vi "Dequeue.vi"(6 "timeout in ms (-1)":i32=-1, 8 "error in (no error)":errorcluster, 11 "Message Queue":T2) -> (0 "error out":errorcluster, 1 "Message Data":variant, 2 "State":T3=enum."Initialize", 3 "Message Queue dub":T2, 4 "# elements in queue":i32, 5 "Caller Info":T1)   [LabVIEW 2019, in "Test.lvlib"]
doc: "This VI pulls messages off the Message Queue."
uses:
  Test.lvlib
  State Name.ctl
  Support/Shared/TypeDefs/Message Queue Ref.ctl
  85968e22-cec5-4834-9408-c5f0918d029d.vi
  0e969a01-278a-410f-94a4-bde872eff04a.vi
  <vilib>/Utility/error.llb/Clear Errors.vi
  <vilib>/Utility/error.llb/Error Cluster From Error Code.vi
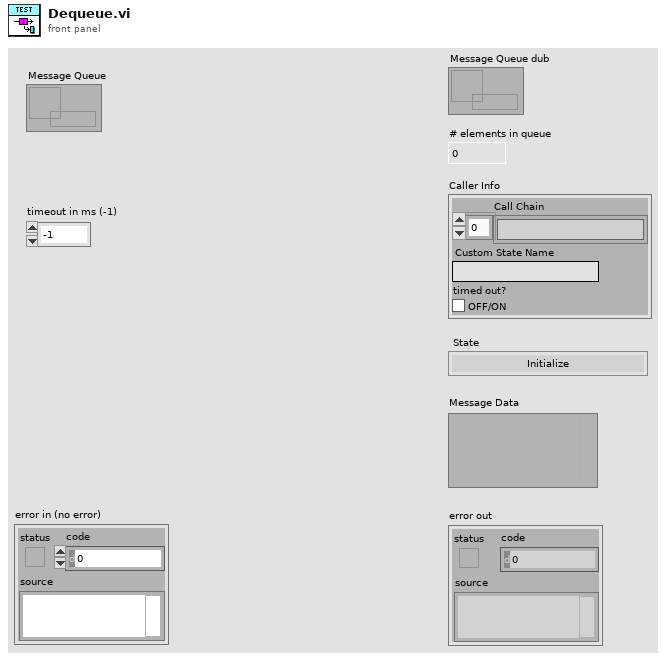
[diagram p1: front panel]
types:
  T1 = cluster{"Call Chain":string[], "Custom State Name":string, "timed out?":bool}
  T2 = typedef "Message Queue Ref.ctl" = refnum<queue>
  T3 = typedef "Test.lvlib/State Name.ctl" = enum16{"Default", "Initialize", "Re-Initialize", "Initialize Data", "Initialize Panel", "[Event Structure] Update Data", "Error", "Exit"}
  T4 = enum16{"Default", "Show FP", "Hide FP", "New Data", "Get Data"}
  T5 = cluster{"Module":string, "State Name":string, "State Dequeue Time":string, "Interval":string, "Call Chain":string, "# elements in queue":i32}
  T6 = cluster{"Call Chain":string[], "Desired State Name":string, "timed out?":bool}
  T7 = cluster{"Custom State Name":string, "Defined State Name":variant, "Call Chain":string[], "Message Data":variant}
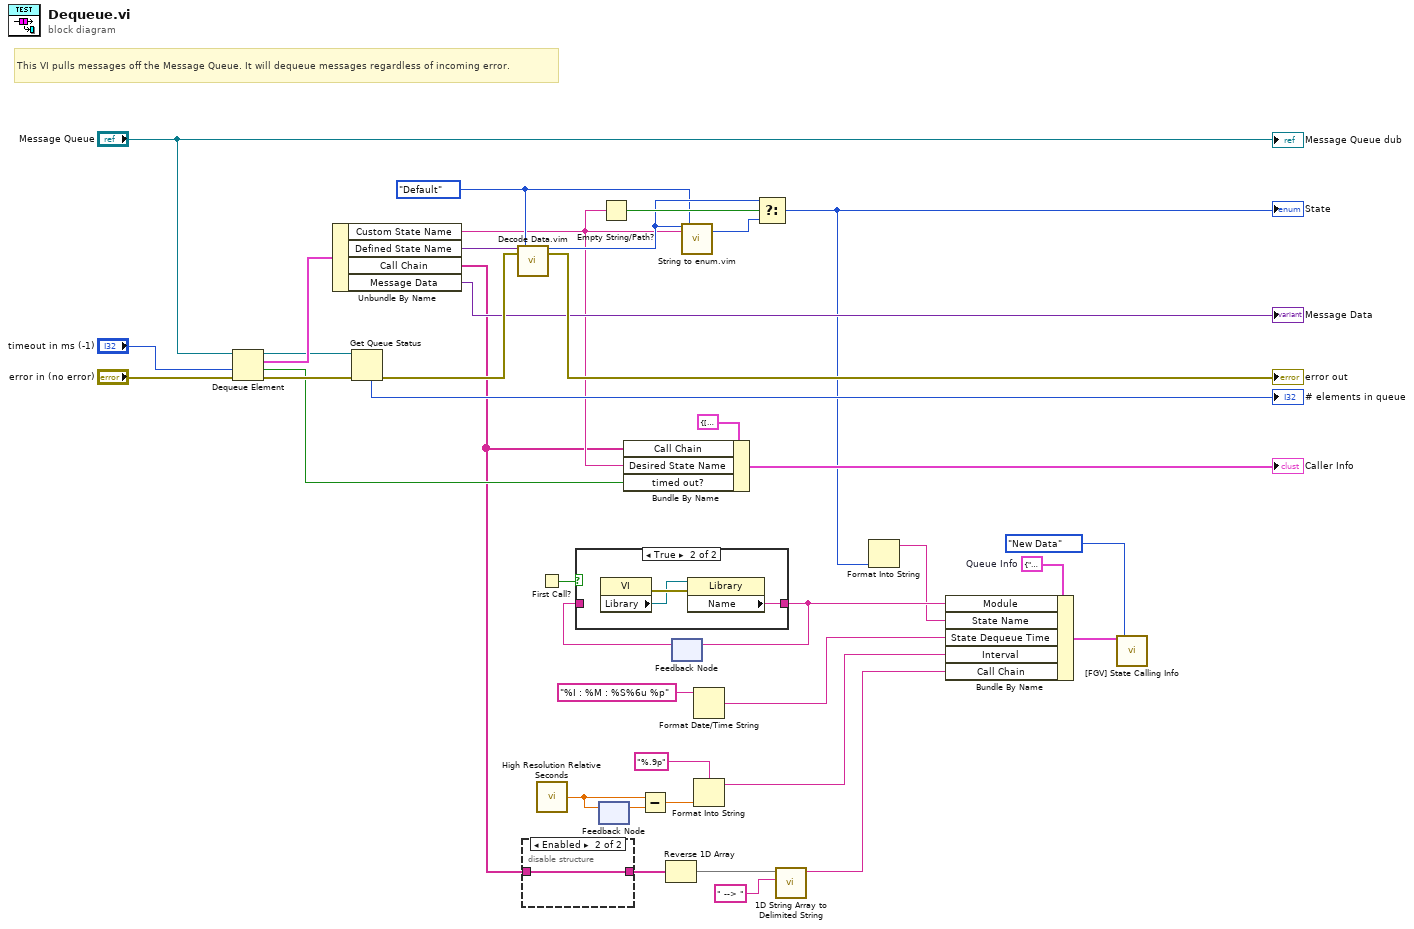
[diagram p0: block diagram]
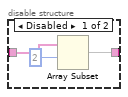
[diagram p2: hidden frame]
diagram:
  w9 = T5 {"Module"="", "State Name"="", "State Dequeue Time"="", "Interval"="", "Call Chain"="", "# elements in queue"=0}  # Queue Info
  w25 = State_Name."Default" ("State")
  # "This VI pulls messages off the Message Queue. It will dequeue messages regardless of incoming error."
  n1 = Dequeue Element(queue="Message Queue", timeout in ms (-1)="timeout in ms (-1)", error in (no error)="error in (no error)") -> (queue out=w37:T2, element=w39:T7, timed out?=w23:bool, error out=w35:errorcluster)
  n2 = Unbundle By Name(w39) -> ("Custom State Name"=w22:string, "Defined State Name"=w32:variant, "Call Chain"=w12:string[], "Message Data"=→"Message Data":variant)
  n3 = Get Queue Status(queue=w37, error in (no error)=w35) -> (error out=w31:errorcluster, # elements in queue=→"# elements in queue":i32)  [unwired: 1 in, 6 out]
  n4 = call "Decode Data.vim"("Data"=w32, "error in"=w31, "Type/Default value"=w25) -> ("Data out"=w26:T3, "error out"=→"error out":errorcluster)  [unwired: 15 in]
  n5 = disable-structure shown="Enabled" {
    disable-tunnel: [w42 w43] -> w13
    disable-tunnel: w12 -> [w40 w43]
    frame Disabled {
      n6 = Array Subset(array=w40, index=2) -> (w42:string[])  [unwired: 1 in]
    }
    frame Enabled {
    }
  }
  n7 = First Call?() -> (First Call?: T/F=w11:bool)
  n8 = call <vilib>:"High Resolution Relative Seconds.vi"() -> ("relative seconds"=w16:dbl)
  n9 = feedback #1() -> (w19:dbl)  [unwired: 1 in]
  n10 = feedback-in #1(w16) -> ()
  n11 = Empty String/Path?(string/path=w22) -> (empty?=w27:bool)
  n12 = Bundle By Name(cluster=T6 {"Call Chain"=[], "Desired State Name"="", "timed out?"=FALSE}, "Call Chain"=w12, "Desired State Name"=w22, "timed out?"=w23) -> (→"Caller Info":T6)
  n13 = Subtract(x=w16, y=w19) -> (x-y=w18:dbl)
  n14 = Reverse 1D Array(array=w13) -> (reversed array=w14:string[])
  n15 = feedback #2() -> (w10:string)  [unwired: 1 in]
  n16 = case shown="True" w11 {
    tunnel: [w44 w45] -> w8
    tunnel: w10 -> [w44 _]
    frame False {
    }
    frame True {
      n17 = property class="VI"() -> (error out=w47:errorcluster, "Library"=w46:refnum<vi>)  [unwired: 2 in, 1 out]
      n18 = property class="Library"(reference=w46, error in=w47) -> ("Name"=w45:string)  [unwired: 2 out]
    }
  }
  n19 = feedback-in #2(w8) -> ()
  n20 = call "String to enum.vim"("Enum"=w26, "Item Name"=w22, "Default Item Name"=w25) -> ("Enum Selected"=w28:T3)  [unwired: 14 in, 2 out]
  n21 = Format Date/Time String(time format string (%c)="%I : %M : %S%6u %p") -> (date/time string=w5:string)  [unwired: 2 in]
  n22 = Format Into String(format string="%.9p", w18) -> (resulting string=w4:string)  [unwired: 2 in, 1 out]
  n23 = Select(t=w26, s=w27, f=w28) -> (s? t:f=w7:T3)
  "State" <- w7
  n24 = call <vilib>:"1D String Array to Delimited String.vi"("delimiter"=" --> ", "string array"=w14) -> ("delimited string"=w3:string)  [unwired: 9 in]
  n25 = Format Into String(w7) -> (resulting string=w6:string)  [unwired: 3 in, 1 out]
  n26 = Bundle By Name(cluster=w9, "Module"=w8, "State Name"=w6, "State Dequeue Time"=w5, "Interval"=w4, "Call Chain"=w3) -> (w2:T5)
  n27 = call "[FGV] State Calling Info.vi"("Queue Info Set"=w2, "Action"=T4."New Data") -> ()  [unwired: 15 in, 3 out]
  "Message Queue dub" <- "Message Queue"
